vi "GetRotation.vi"(3 "Az":dbl, 4 "Ay":dbl, 5 "Ax":dbl) -> (0 "Yaw":dbl, 1 "Pitch":dbl, 2 "Roll":dbl)   [LabVIEW 2011]
uses:
  <vilib>/express/express arith-compare/Formula/XNode/ExpressFormulaBlockNode.xnode
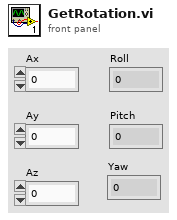
[diagram p1: front panel]
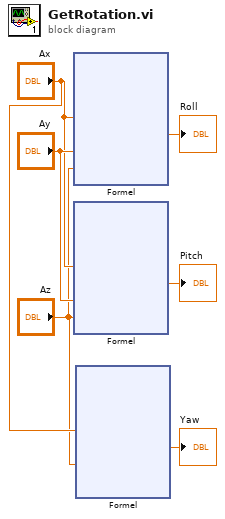
[diagram p0: block diagram]
diagram:
  n1 = xnode "Formel"("Ax"="Ax", "Ay"="Ay", "Az"="Az") -> ("Ergebnis"=→"Roll":dbl)  [unwired: 1 in, 1 out]
  n2 = xnode "Formel"("Ax"="Ax", "Ay"="Ay", "Az"="Az") -> ("Ergebnis"=→"Pitch":dbl)  [unwired: 1 in, 1 out]
  n3 = xnode "Formel"("Ax"="Ax", "Az"="Az") -> ("Ergebnis"=→"Yaw":dbl)  [unwired: 2 in, 1 out]
